vi "PH_Tektronix_7000.IDN.vi"(0 "i ref in":refnum<vi>, 5 "error IO":errorcluster) -> (14 "i ref out":refnum<vi>, 19 "error out":errorcluster)   [LabVIEW 2014, in "PH_Tektronix_7000.lvlib"]
doc: "If the connection is established, this VI queries several informations from the instrument."
uses:
  PH_Tektronix_7000.lvlib
  non_GPL/instr.lib/Tektronix 7000 Series/Tektronix 7000 Series - Driver np.lvlib
  PH_Common/PH_Common.lvlib
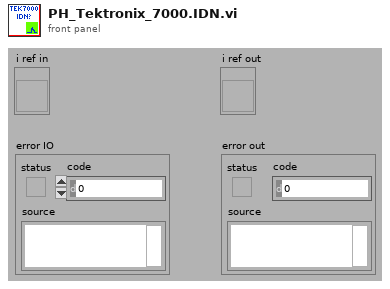
[diagram p1: front panel]
types:
  T1 = typedef "PH_Tektronix_7000.lvlib/PH_Tektronix_7000.i attribute.ctl" = cluster{"VISA Resource Name":refnum<visa-resource-name>, "IDN":cluster{"Instrument Driver":string, "Instrument Firmware":string, "Model":string, "Serial Number":string}, "Selftest":cluster{"Result":i32, "Message":string}, "Trigger Configuration":T2, "Acquisition Configuration":T3, "GUI Refs":T4, "State":T5, "Error Message":string, "Allow Prdc Loop?":bool, "Channel 1":T6, "Channel 2":T6, "Channel 3":T6, "Channel 4":T6, "Data CH 1":waveform(dbl), "Data CH 2":waveform(dbl), "Data CH 3":waveform(dbl), "Data CH 4":waveform(dbl), "Allow config?":bool, "Name Channel 1":string, "Name Channel 2":string, "Name Channel 3":string, "Name Channel 4":string, "Fetch Data before sending to PSDB?":bool, "Constructor passed?":bool, "Data taken at":timestamp, "Plot Colors":u32[], "Default VISA Resource":string}
  T2 = typedef "PH_Tektronix_7000.lvlib/PH_Tektronix_7000.Trigger Config.ctl" = cluster{"Source":u16, "Level [V]":dbl, "Slope":u16, "Coupling":u16, "Trigger Mode":u16}
  T3 = typedef "PH_Tektronix_7000.lvlib/PH_Tektronix_7000.Acquisition Config.ctl" = cluster{"Record Length":u32, "Timebase [s/div]":dbl, "Position [%]":dbl, "Acquisition Type":u16, "Average Waveforms":i32, "Envelope Waveforms":i32, "WfmDB Samples":i32, "Continuous?":bool, "Delay [s]":dbl, "Run?":bool}
  T4 = typedef "PH_Tektronix_7000.lvlib/PH_Tektronix_7000.GUI Refs.ctl" = cluster{"Graph":refnum<vi>, "State":refnum<vi>, "Delete":refnum<vi>, "VISA Resource":refnum<vi>, "Allow Configure":refnum<vi>, "Fetch Data":refnum<vi>, "Fetch before sending Data to PSDB":refnum<vi>, "Name Channel 1":refnum<vi>, "Name Channel 2":refnum<vi>, "Name Channel 3":refnum<vi>, "Name Channel 4":refnum<vi>, "Prdc Intervall [ms]":refnum<vi>, "Data taken":refnum<vi>, "Model":refnum<vi>, "Serial Number":refnum<vi>, "Firmware":refnum<vi>, "Driver":refnum<vi>, "Acquisition":refnum<vi>, "Trigger":refnum<vi>, "Cursor: D Time [s]":refnum<vi>, "Cursor: D Signal [V]":refnum<vi>, "Channel 1":refnum<vi>, "Channel 2":refnum<vi>, "Channel 3":refnum<vi>, "Channel 4":refnum<vi>}
  T5 = typedef "PH_StatusHandler.lvlib/PH_StatusHandler.Status.ctl" = i16
  T6 = typedef "PH_Tektronix_7000.lvlib/PH_Tektronix_7000.Channel Config.ctl" = cluster{"Enable Channel":bool, "Bandwidth":u16, "Input Impedance":u16, "Vertical Coupling":u16, "Probe Attenuation":dbl, "Range [V/div]":dbl, "Position [div]":dbl, "Bandwidth raw":string}
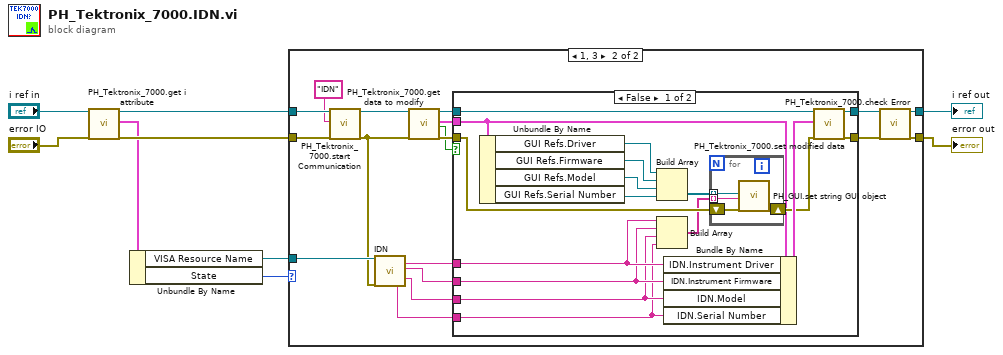
[diagram p0: block diagram]
diagram:
  n1 = call "PH_Tektronix_7000.get i attribute.vi"("i ref in"="i ref in", "error in (no error)"="error IO") -> ("i ref out"=w4:refnum<vi>, "i attribute"=w6:T1, "error out"=w8:errorcluster)  [unwired: 15 in]
  n2 = Unbundle By Name(w6) -> ("VISA Resource Name"=w7:refnum<visa-resource-name>, "State"=w1:T5)
  n3 = case shown="1, 3" w1 {
    tunnel: w4 -> [w11 w15]
    tunnel: w7 -> [_ w24]
    tunnel: w8 -> [w10 w23]
    tunnel: [w11 w19] -> w9
    tunnel: [w10 w17] -> w2
    frame Default {
    }
    frame 1, 3 {
      n4 = call "PH_Tektronix_7000.start Communication.vi"("i ref in"=w15, "Action"="IDN", "error in"=w23) -> ("i ref out"=w16:refnum<vi>, "error out"=w20:errorcluster)  [unwired: 15 in]
      n5 = call "IDN.vi"("VISA resource name"=w24, "error in (no error)"=w20) -> ("Serial Number"=w12:string, "Instrument Driver Revision"=w22:string, "Instrument Firmware Revision"=w21:string, "Model"=w13:string)  [unwired: 11 in, 3 out]
      n6 = call "PH_Tektronix_7000.get data to modify.vi"("i ref in"=w16, "error in (no error)"=w20) -> ("i ref out"=w27:refnum<vi>, "i attribute"=w25:T1, "timed out"=w26:bool, "error out"=w28:errorcluster)  [unwired: 14 in]
      n7 = case shown="False" w26 {
        tunnel: [w46 w51] -> w18
        tunnel: w28 -> [w35 w51]
        tunnel: w27 -> [w45 w52]
        tunnel: [w44 w52] -> w29
        tunnel: w25 -> [w41 _]
        tunnel: w22 -> [w34 _]
        tunnel: w21 -> [w33 _]
        tunnel: w13 -> [w32 _]
        tunnel: w12 -> [w31 _]
        frame False {
          n8 = Unbundle By Name(w41) -> ("GUI Refs.Driver"=w40:refnum<vi>, "GUI Refs.Firmware"=w39:refnum<vi>, "GUI Refs.Model"=w38:refnum<vi>, "GUI Refs.Serial Number"=w37:refnum<vi>)
          n9 = Build Array(w40, w39, w38, w37) -> (w36:refnum<vi>[])
          n10 = Build Array(w34, w33, w32, w31) -> (w30:string[])
          n11 = Bundle By Name(cluster=w41, "IDN.Instrument Driver"=w34, "IDN.Instrument Firmware"=w33, "IDN.Model"=w32, "IDN.Serial Number"=w31) -> (w43:T1)
          n12 = for {
            tunnel: w36 -> [w48] mode=indexing
            shift-right: [w49] -> w42
            shift-left: w35 -> [w50]
            tunnel: w30 -> [w47] mode=indexing
            n13 = call "PH_GUI.set string GUI object.vi"("GUI object Ref"=w48, "Text"=w47, "error in"=w50) -> ("error out"=w49:errorcluster)  [unwired: 16 in]
          }
          n14 = call "PH_Tektronix_7000.set modified data.vi"("i ref in"=w45, "i attribute"=w43, "error in (no error)"=w42) -> ("i ref out"=w44:refnum<vi>, "error out"=w46:errorcluster)  [unwired: 15 in]
        }
        frame True {
        }
      }
      n15 = call "PH_Tektronix_7000.check Error.vi"("i ref in"=w29, "error in"=w18) -> ("i ref out"=w19:refnum<vi>, "error out"=w17:errorcluster)  [unwired: 16 in]
    }
  }
  "i ref out" <- w9
  "error out" <- w2
